vi "SaveData.vi"(8 "error in (no error)":errorcluster, 9 "Comments":string="Comment Thread", 10 "File Name":path, 11 "Synapse CCD.lvclass In":refnum<class "Synapse CCD.lvclass">) -> (0 "error out":errorcluster, 3 "Synapse CCD.lvclass Out":refnum<class "Synapse CCD.lvclass">)   [LabVIEW 2012, in "Synapse CCD.lvclass"]
doc: "Packages Processed and Raw Data for Export to Excel.vi"
uses:
  Synapse CCD.lvclass
  Synapse CCD.lvclass/Synapse CCD.ctl
  Utility Classes/Readable/Readable.lvclass
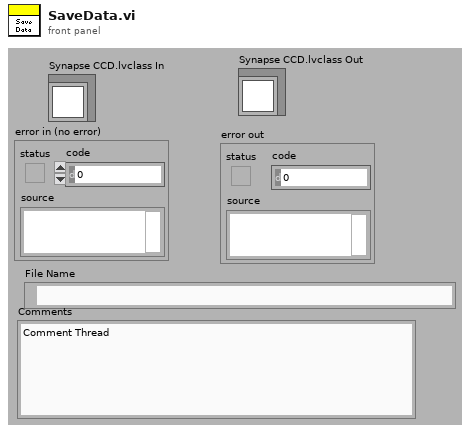
[diagram p1: front panel]
types:
  T1 = typedef "Readable.lvclass/Channel Names.ctl" = string[]
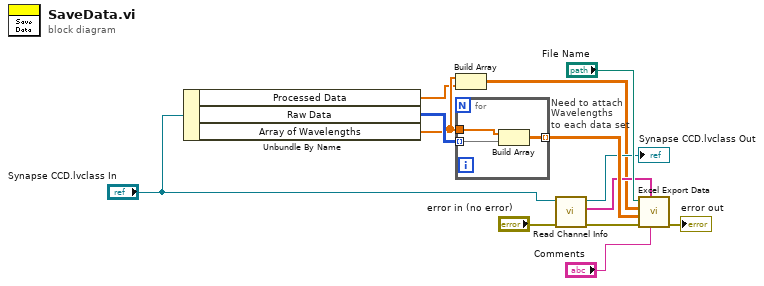
[diagram p0: block diagram]
diagram:
  n1 = Unbundle By Name("Synapse CCD.lvclass In") -> ("Processed Data"=w8:dbl[], "Raw Data"=w11:i32[][], "Array of Wavelengths"=w9:dbl[])
  n2 = Build Array(w9, w8) -> (w1:dbl[][])
  n3 = for "Need to attach Wavelengths\nto each data set" {
    tunnel: w11 -> [w15] mode=indexing
    tunnel: w9 -> [w16]
    tunnel: [w14] -> w10 mode=indexing
    n4 = Build Array(w16, w15) -> (w14:dbl[][])
  }
  n5 = call "Read Channel Info.vi"("error in (no error)"="error in (no error)", "Readable.lvclass in"="Synapse CCD.lvclass In") -> ("error out"=w2:errorcluster, "Channel Names"=w4:T1, "Readable.lvclass out"=→"Synapse CCD.lvclass Out":refnum<class "Synapse CCD.lvclass">)  [unwired: 5 in, 2 out]
  n6 = call "Excel Export Data.vi"("Comments"="Comments", "Channel Names"=w4, "error in (no error)"=w2, "Raw Data"=w10, "Processed Data"=w1, "File Name"="File Name") -> ("error out"=→"error out":errorcluster)  [unwired: 5 in]
